vi "set Value.vi"(8 "error in (no error)":errorcluster, 10 "Value":variant, 11 "AISAS motor in":refnum<class "AISAS motor.lvclass">) -> (0 "error out":errorcluster, 3 "AISAS motor out":refnum<class "AISAS motor.lvclass">)   [LabVIEW 2014, in "AISAS motor.lvclass"]
uses:
  AISAS motor.lvclass
  AISAS motor.lvclass/AISAS motor.ctl
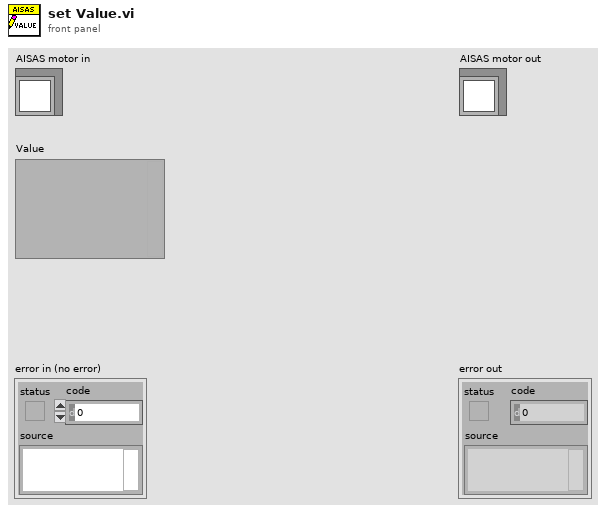
[diagram p1: front panel]
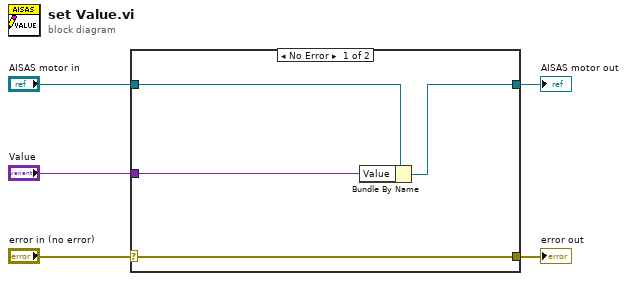
[diagram p0: block diagram]
diagram:
  n1 = case shown="No Error" "error in (no error)" {
    selector: "error in (no error)" -> [w9 w10]
    tunnel: [w9 w10] -> w4
    tunnel: [w7 w11] -> w2
    tunnel: "AISAS motor in" -> [w8 w11]
    tunnel: "Value" -> [w6 _]
    frame No Error {
      n2 = Bundle By Name(cluster=w8, "Value"=w6) -> (w7:refnum<class "AISAS motor.lvclass">)
    }
    frame Error {
    }
  }
  "error out" <- w4
  "AISAS motor out" <- w2
